vi "Get UI Details.vi"() -> ()   [LabVIEW 2021, in "audio_adc_acDualChannelMeasurement.lvlib"]
uses:
  audio_adc_acDualChannelMeasurement.lvlib
  <vilib>/MeasurementLink/MeasurementLink Measurement Server/Helpers/TypeDefs/UI Information.ctl
  <vilib>/MeasurementLink/MeasurementLink Measurement Server/MeasurementLink Measurement Server.lvlib
panel:
  out "error out":errorcluster
  in  "error in (no error)":errorcluster
  out "UI Details":T1[](array[typedef])
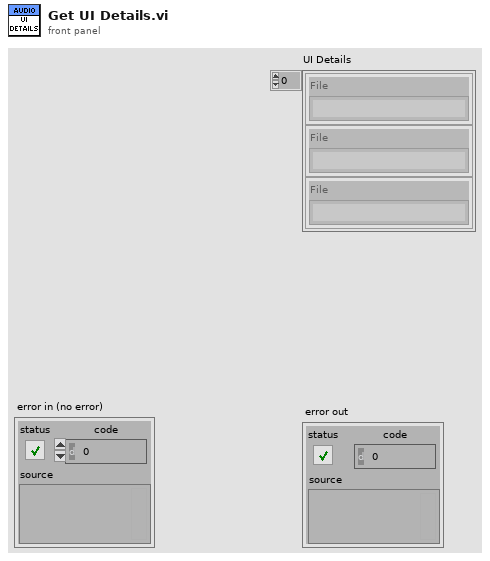
[diagram p1: front panel]
types:
  T1 = typedef "MeasurementLink Measurement Server.lvlib/UI Information.ctl" = cluster{"File":string}
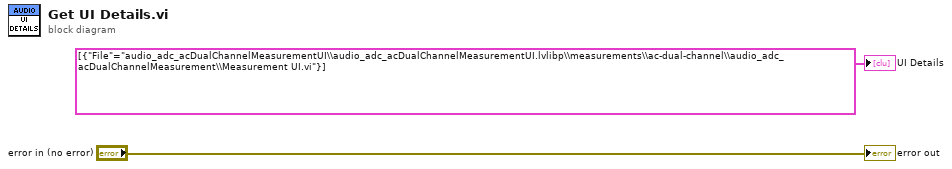
[diagram p0: block diagram]
diagram:
  "UI Details" <- T1[] [{"File"="audio_adc_acDualChannelMeasurementUI\\audio_adc_acDualChannelMeasurementUI.lvlibp\\measurements\\ac-dual-channel\\audio_adc_acDualChannelMeasurement\\Measurement UI.vi"}] ("UI Details")
  "error out" <- "error in (no error)"
